vi "Implement When VIs.vi"(8 "error in (no error)":errorcluster, 10 "When VIs":path[](array[path]), 11 "Mock Class Generator In":refnum<class "Pure Mock Class Generator.lvclass">) -> (0 "error out":errorcluster, 3 "Mock Class Generator Out":refnum<class "Pure Mock Class Generator.lvclass">)   [LabVIEW 2020]
uses:
  Pure Mock Class Generator.lvclass
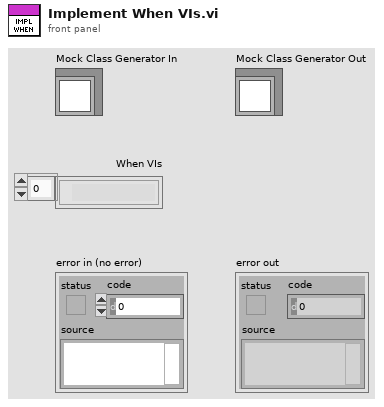
[diagram p1: front panel]
types:
  T1 = enum16{"Invalid Wire Rule", "Required", "Recommended", "Optional", "Dynamic Dispatch"}
  T2 = enum16{"Invalid Wire Rule", "Required", "Recommended", "Optional", "Dynamic Dispatch"}[]
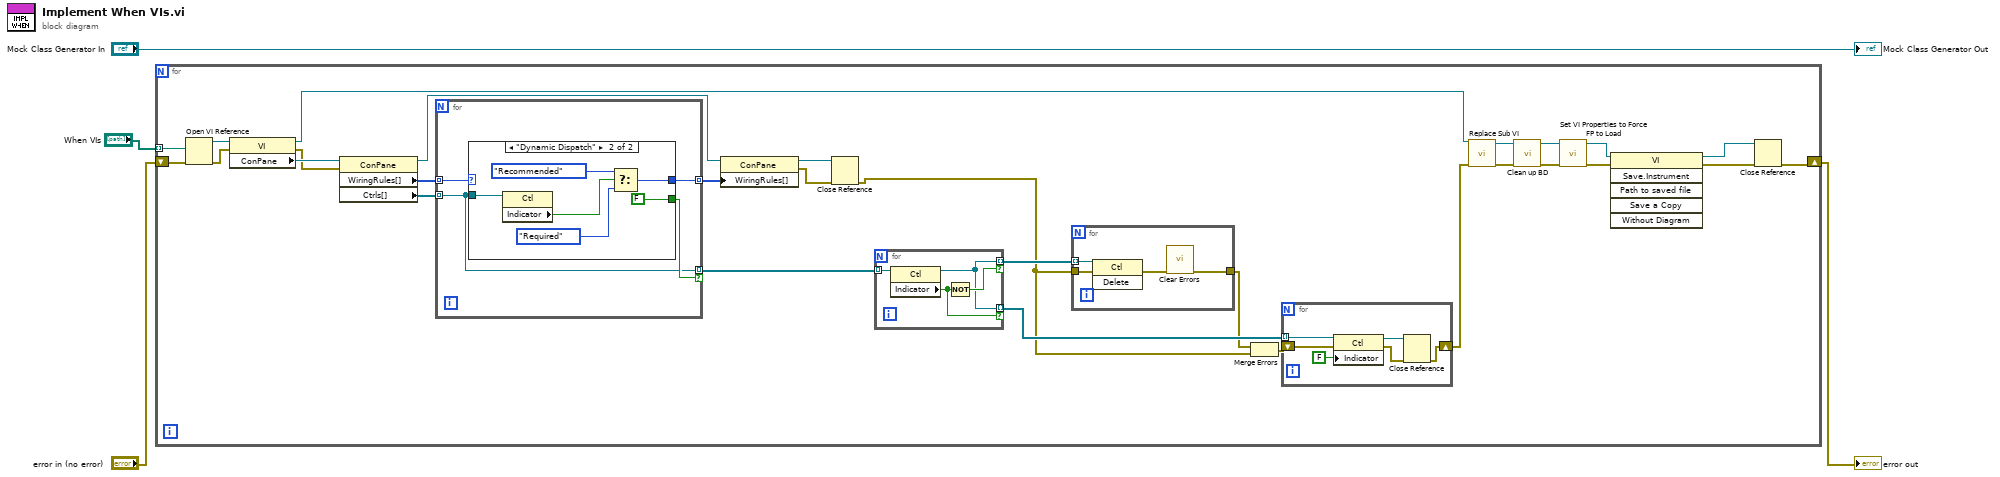
[diagram p0: block diagram]
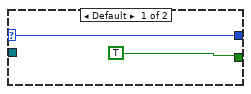
[diagram p2: hidden frame]
diagram:
  n1 = for {
    tunnel: "When VIs" -> [w33] mode=indexing
    shift-right: [w18] -> w1
    shift-left: "error in (no error)" -> [w32]
    n2 = Open VI Reference(vi path=w33, error in (no error)=w32) -> (vi reference=w31:refnum<vi>, error out=w23:errorcluster)  [unwired: 4 in]
    n3 = property class="VI"(reference=w31, error in=w23) -> (reference out=w19:refnum<vi>, error out=w20:errorcluster, "ConPane"=w30:refnum<vi>)
    n4 = property class="ConPane"(reference=w30, error in=w20) -> (reference out=w26:refnum<vi>, "WiringRules[]"=w29:T2, "Ctrls[]"=w27:refnum<vi>[])  [unwired: 1 out]
    n5 = for {
      tunnel: w29 -> [w37] mode=indexing
      tunnel: [w36] -> w28 mode=indexing
      tunnel: w27 -> [w34] mode=indexing
      tunnel: [w34] -> w25 mode=indexing if=w35
      n6 = case shown="\"Dynamic Dispatch\"" w37 {
        selector: w37 -> [w39 _]
        tunnel: [w39 w42] -> w36
        tunnel: [TRUE FALSE] -> w35
        tunnel: w34 -> [_ w43]
        frame Default {
        }
        frame "Dynamic Dispatch" {
          n7 = property class="Ctl"(reference=w43) -> ("Indicator"=w41:bool)  [unwired: 1 in, 2 out]
          n8 = Select(t=T1."Recommended" ("Wire Rule"), s=w41, f=T1."Required" ("Wire Rule")) -> (s? t:f=w42:T1)
        }
      }
    }
    n9 = property class="ConPane"(reference=w26, "WiringRules[]"=w28) -> (reference out=w10:refnum<vi>, error out=w22:errorcluster)  [unwired: 1 in]
    n10 = Close Reference(reference=w10, error in (no error)=w22) -> (error out=w11:errorcluster)
    n11 = for {
      tunnel: [w57] -> w24 mode=indexing if=w58
      tunnel: w25 -> [w59] mode=indexing
      tunnel: [w57] -> w21 mode=indexing if=w56
      n12 = property class="Ctl"(reference=w59) -> (reference out=w57:refnum<vi>, "Indicator"=w56:bool)  [unwired: 1 in, 1 out]
      n13 = Not(x=w56) -> (.not. x?=w58:bool)
    }
    n14 = for {
      tunnel: w24 -> [w55] mode=indexing
      tunnel: w11 -> [w53]
      tunnel: [w52] -> w13
      n15 = invoke class="Ctl" method="Delete"(reference=w55, error in=w53) -> (error out=w54:errorcluster)  [unwired: 1 in, 2 out]
      n16 = call <vilib>:"Clear Errors.vi"("error in (no error)"=w54) -> ("error out"=w52:errorcluster)  [unwired: 5 in, 1 out]
    }
    n17 = Merge Errors(w13, w11) -> (w12:errorcluster)
    n18 = for {
      tunnel: w21 -> [w51] mode=indexing
      shift-right: [w46] -> w17
      shift-left: w12 -> [w47]
      n19 = property class="Ctl"(reference=w51, error in=w47, "Indicator"=FALSE) -> (reference out=w48:refnum<vi>, error out=w49:errorcluster)
      n20 = Close Reference(reference=w48, error in (no error)=w49) -> (error out=w46:errorcluster)
    }
    n21 = call "Replace Sub VI.vi"("error in (no error)"=w17, "VI in"=w19) -> ("error out"=w16:errorcluster, "VI out"=w6:refnum<vi>)  [unwired: 8 in]
    n22 = call "Clean up BD.vi"("error in (no error)"=w16, "VI in"=w6) -> ("error out"=w7:errorcluster, "VI out"=w5:refnum<vi>)  [unwired: 8 in]
    n23 = call "Set VI Properties to Force FP to Load.vi"("error in (no error)"=w7, "VI in"=w5) -> ("error out"=w9:errorcluster, "VI out"=w8:refnum<vi>)  [unwired: 8 in]
    n24 = invoke class="VI" method="Save.Instrument"(reference=w8, error in=w9) -> (reference out=w14:refnum<vi>, error out=w15:errorcluster)  [unwired: 4 in, 4 out]
    n25 = Close Reference(reference=w14, error in (no error)=w15) -> (error out=w18:errorcluster)
  }
  "error out" <- w1
  "Mock Class Generator Out" <- "Mock Class Generator In"
